vi "Initialize - Set Configuration File.vi"(8 "error in (no error)":errorcluster, 9 "Export to File on Save":refnum<vi>, 10 "Export Path":refnum<vi>, 11 "Item Ref in":T1 format="%.0x") -> (0 "error out":errorcluster, 3 "Item Ref out":T1 format="%.0x")   [LabVIEW 2019, in "UDP-Custom-Device System Explorer.lvlib"]
doc: "Sets the <b>Export to File Status</b> and <b>Export File</b> based on their associated page properties."
uses:
  UDP-Custom-Device System Explorer.lvlib
  <vilib>/NI VeriStand/Custom Device API/Custom Device Item Ref.ctl
  Property Accessors/Main Accessors.lvlib
  <vilib>/NI VeriStand/Custom Device API/Custom Device API.lvlib
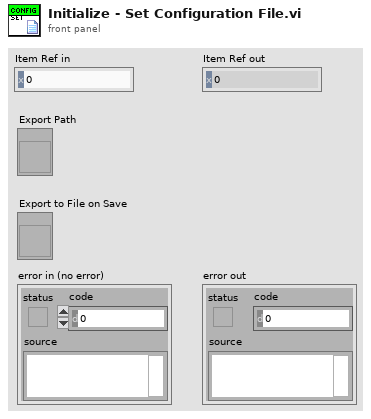
[diagram p1: front panel]
types:
  T1 = typedef "Custom Device API.lvlib/Custom Device Item Ref.ctl" = u64
  T2 = enum8{"Enabled", "Disabled", "Disabled and Grayed Out"}
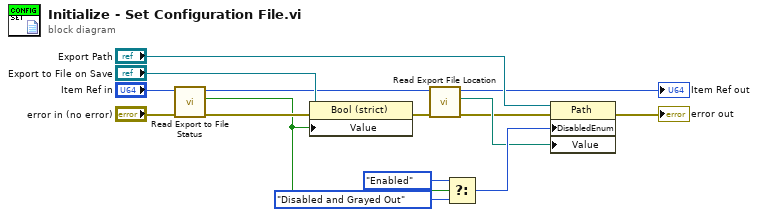
[diagram p0: block diagram]
diagram:
  n1 = call "Read Export to File Status.vi"("error in (no error)"="error in (no error)", "Node Ptr"="Item Ref in") -> ("error out"=w7:errorcluster, "Export to File Status"=w6:bool, "Node Ptr out"=w4:T1)  [unwired: 7 in]
  n2 = property class="Bool (strict)"(reference="Export to File on Save", error in=w7, "Value"=w6) -> (error out=w5:errorcluster)  [unwired: 1 out]
  n3 = call "Read Export File Location.vi"("error in (no error)"=w5, "Node Ptr"=w4) -> ("error out"=w1:errorcluster, "Export File Location"=w2:path, "Node Ptr out"=→"Item Ref out":T1)  [unwired: 7 in]
  n4 = Select(t=T2."Enabled" ("Disabled"), s=w6, f=T2."Disabled and Grayed Out" ("Disabled")) -> (s? t:f=w14:T2)
  n5 = property class="Path"(reference="Export Path", error in=w1, "DisabledEnum"=w14, "Value"=w2) -> (error out=→"error out":errorcluster)  [unwired: 1 out]
